vi "Normalize_subvi.vi"(1 "Y":dbl[](array[numeric])) -> (0 "Array":dbl[](array[numeric]))   [LabVIEW 2020]
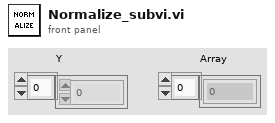
[diagram p1: front panel]
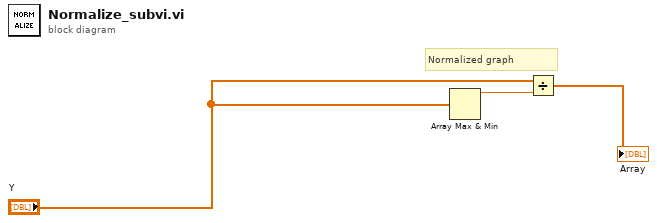
[diagram p0: block diagram]
diagram:
  # "Normalized graph"
  n1 = Array Max & Min(array="Y") -> (max value=w2:dbl)  [unwired: 3 out]
  n2 = Divide(x="Y", y=w2) -> (x/y=→"Array":dbl[])
